vi "List Blob Snapshots.vi"(8 "error in (no error)":errorcluster, 9 "Blob name":string, 10 "Container":string, 11 "Azure Session in":refnum<class "Session.lvclass">) -> (0 "error out":errorcluster, 2 "Blob snapshots":string[](array[string]), 3 "Azure Session out":refnum<class "Session.lvclass">)   [LabVIEW 2015, in "NI_Azure_Blob.lvlib"]
doc: "Lists all snapshots of a blob."
uses:
  NI_Azure_Blob.lvlib
  Core/Session/Session.lvclass
  Core/Name Value Pair.ctl
  Core/Session/Session.lvclass/Session.ctl
  Core/Session/Write Request Parameters.vi
  Core/Session/Write HTTP Verb.vi
  Core/Session/Write URL Suffix.vi
  Core/NI_Azure_Core.lvlib
  XML Parsing/NI_Azure_XML Parsing.lvlib
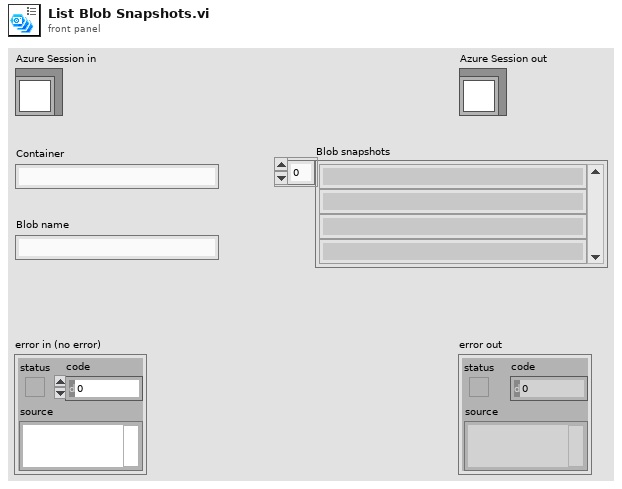
[diagram p1: front panel]
types:
  T1 = typedef "NI_Azure_Core.lvlib/Name Value Pair.ctl" = cluster{"name":string, "value":string}
  T2 = typedef "NI_Azure_Core.lvlib/Response.ctl" = cluster{"Headers":string, "Body":string}
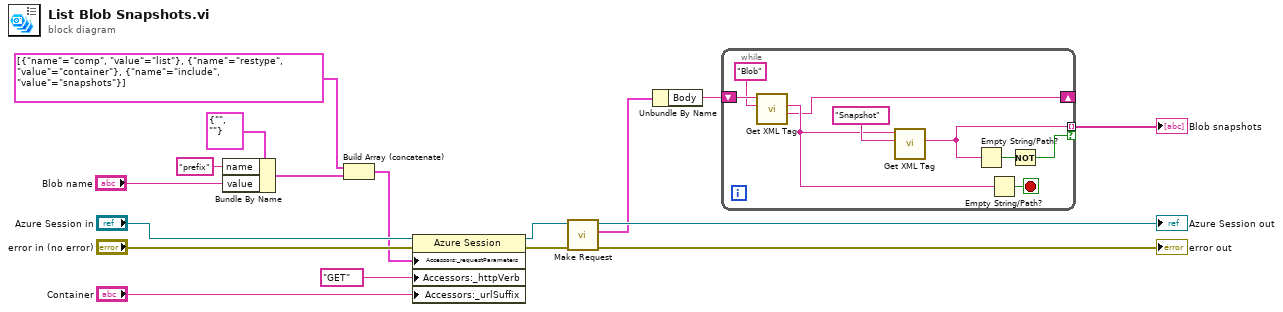
[diagram p0: block diagram]
diagram:
  n1 = Bundle By Name(cluster=T1 {"name"="", "value"=""} ("Name Value Pair"), "name"="prefix", "value"="Blob name") -> (w4:T1)
  n2 = Build Array (concatenate)(T1[] [{"name"="comp", "value"="list"}, {"name"="restype", "value"="container"}, {"name"="include", "value"="snapshots"}] ("request parameters"), w4) -> (w2:T1[])
  n3 = property class="Azure Session"(reference="Azure Session in", error in="error in (no error)", "Accessors:_requestParameters"=w2, "Accessors:_httpVerb"="GET" ("HTTP-Verb"), "Accessors:_urlSuffix"="Container") -> (reference out=w9:refnum<class "Session.lvclass">, error out=w11:errorcluster)
  n4 = call "Make Request.vi"("error in (no error)"=w11, "Session in"=w9) -> ("error out"=→"error out":errorcluster, "Response"=w12:T2, "Session out"=→"Azure Session out":refnum<class "Session.lvclass">)  [unwired: 7 in]
  n5 = Unbundle By Name(w12) -> ("Body"=w13:string)
  n6 = while {
    shift-right: [w21] -> _
    shift-left: w13 -> [w26]
    tunnel: [w20] -> w14 mode=indexing if=w18
    stop <- w24 stop-if-true
    n7 = call "Get XML Tag.vi"("Tag name"="Blob", "XML String in"=w26) -> ("Remaining string"=w21:string, "Tag value"=w22:string)  [unwired: 5 in, 3 out]
    n8 = call "Get XML Tag.vi"("Tag name"="Snapshot", "XML String in"=w22) -> ("Tag value"=w20:string)  [unwired: 5 in, 4 out]
    n9 = Empty String/Path?(string/path=w20) -> (empty?=w19:bool)
    n10 = Empty String/Path?(string/path=w22) -> (empty?=w24:bool)
    n11 = Not(x=w19) -> (.not. x?=w18:bool)
  }
  "Blob snapshots" <- w14
